vi "thermocoupleMain.vi"() -> ()   [LabVIEW 2023]
uses:
  <vilib>/Utility/file.llb/Write Delimited Spreadsheet (DBL).vi
  <vilib>/Analysis/NI_AALBase.lvlib
panel:
  out "temperature 2":dbl format="%0.2f"
  out "standard deviation":dbl format="%0.2f"
  out "mean":dbl format="%0.6e"
  in  "Below 0":bool
  in  "file path (dialog if empty)":path
  in  "stop":bool
  in  "V0(for0degC)":dbl=-0.00072 format="%#_13g"
  out "Temperature (deg C)":dbl(graph)
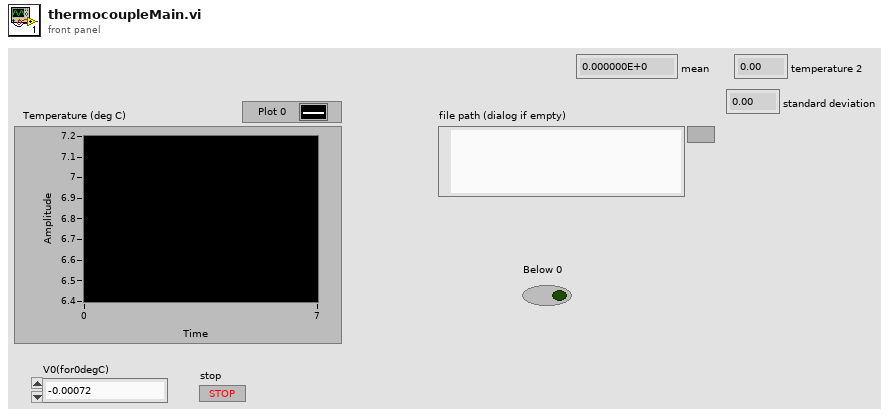
[diagram p1: front panel]
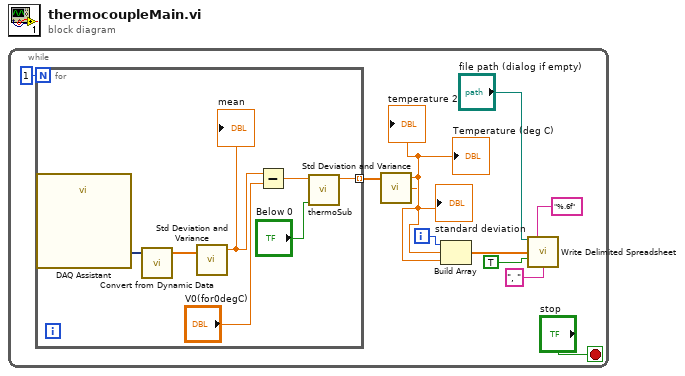
[diagram p0: block diagram]
diagram:
  n1 = while {
    i -> [w10]
    stop <- "stop" stop-if-true
    n2 = for {
      N: 1 -> [_]
      tunnel: [w12] -> w5 mode=indexing
      n3 = call "DAQ Assistant"() -> ("data"=w18:dynamicdata)  [unwired: 17 in, 2 out]
      n4 = call "Convert from Dynamic Data"("Dynamic Data Type"=w18) -> ("Array"=w17:dbl[])  [unwired: 3 in]
      n5 = call <vilib>:"Std Deviation and Variance.vi"("X"=w17) -> ("mean"=w15:dbl)  [unwired: 1 in, 2 out]
      "mean" <- w15
      n6 = Subtract(x=w15, y="V0(for0degC)") -> (x-y=w13:dbl)
      n7 = call "thermoSub.vi"("Below 0?"="Below 0", "Voltage(mV)"=w13) -> ("output variable"=w12:dbl)  [unwired: 9 in]
    }
    n8 = call <vilib>:"Std Deviation and Variance.vi"("X"=w5) -> ("mean"=w4:dbl, "standard deviation"=w3:dbl)  [unwired: 1 in, 1 out]
    "Temperature (deg C)" <- w4
    "standard deviation" <- w3
    "temperature 2" <- w4
    n9 = Build Array(w10, w4, w3) -> (w9:dbl[])
    n10 = call-poly <vilib>:"Write Delimited Spreadsheet.vi"("file path (dialog if empty)"="file path (dialog if empty)", "format (%.3f)"="%.6f", "1D data"=w9, "append to file? (new file:F)"=TRUE, "delimiter (\\t)"=", " ("delimiter (\\t)")) -> ()  [unwired: 9 in, 2 out]
  }
